vi "angleToDistance.vi"(9 "Angle":dbl, 10 "Length":dbl, 11 "Width":dbl) -> (3 "zDistance":dbl)   [LabVIEW 2017]
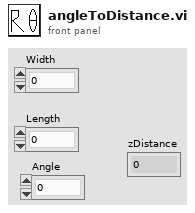
[diagram p1: front panel]
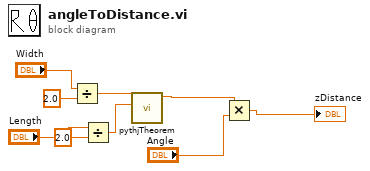
[diagram p0: block diagram]
diagram:
  n1 = Divide(x="Width", y=2.0) -> (x/y=w5:dbl)
  n2 = Divide(x="Length", y=2.0) -> (x/y=w4:dbl)
  n3 = call "pythjTheorem.vi"("yDistance"=w4, "xDistance"=w5) -> ("autoDistance"=w3:dbl)  [unwired: 9 in]
  n4 = Multiply(x=w3, y="Angle") -> (x*y=→"zDistance":dbl)
